vi "Add default dependencies.vi"(8 "error in (no error)":errorcluster, 11 "Targets in":refnum<class "Targets.lvclass">) -> (0 "error out":errorcluster, 3 "Targets out":refnum<class "Targets.lvclass">)   [LabVIEW 2013, in "PL Framework Configuration Tool.lvlib" / "Targets.lvclass"]
uses:
  Targets.lvclass
  Targets.lvclass/Targets.ctl
  TBM Configuration Node/deployment configuration.ctl
  TBM Configuration Node/TBM Configuration Node.lvclass
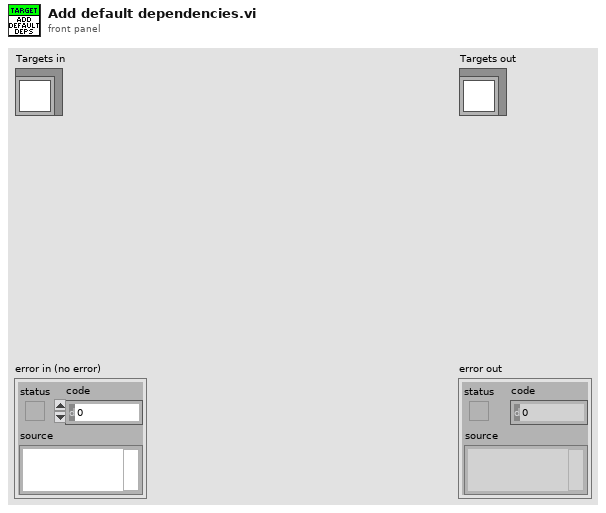
[diagram p1: front panel]
types:
  T1 = typedef "PL Framework Configuration Tool.lvlib/TBM Configuration Node.lvclass/deployment configuration.ctl" = cluster{"local path":path, "remote path (relative to root)":path}
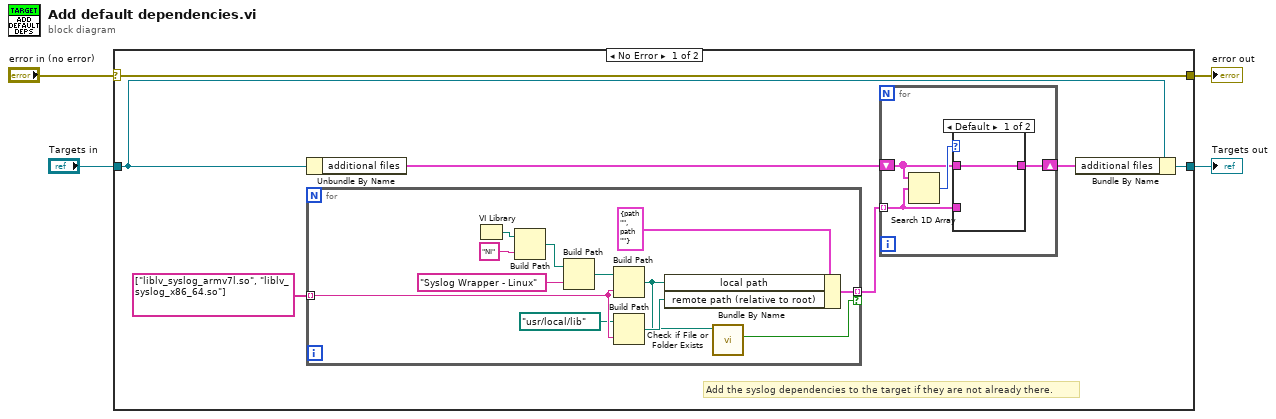
[diagram p0: block diagram]
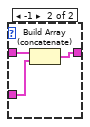
[diagram p2: hidden frame]
diagram:
  n1 = case shown="No Error" "error in (no error)" {
    selector: "error in (no error)" -> [w11 w33]
    tunnel: [w11 w33] -> w3
    tunnel: [w8 w32] -> w1
    tunnel: "Targets in" -> [w9 w32]
    frame No Error {
      # "Add the syslog dependencies to the target if they are not already there."
      n2 = Unbundle By Name(w9) -> ("additional files"=w7:T1[])
      n3 = for {
        tunnel: string[] ["liblv_syslog_armv7l.so", "liblv_syslog_x86_64.so"] -> [w24] mode=indexing
        tunnel: [w23] -> w6 mode=indexing if=w21
        n4 = VI Library() -> (path=w30:path)
        n5 = Build Path(base path=w30, name or relative path="NI") -> (appended path=w28:path)
        n6 = Build Path(base path=w28, name or relative path="Syslog Wrapper - Linux") -> (appended path=w26:path)
        n7 = Build Path(base path=w26, name or relative path=w24) -> (appended path=w22:path)
        n8 = Build Path(base path=path "/usr/local/lib", name or relative path=w24) -> (appended path=w25:path)
        n9 = Bundle By Name(cluster=T1 {"local path"=path "", "remote path (relative to root)"=path ""} ("deployment configuration"), "local path"=w22, "remote path (relative to root)"=w25) -> (w23:T1)
        n10 = call <vilib>:"Check if File or Folder Exists.vi"("path"=w22) -> ("file or folder exists?"=w21:bool)  [unwired: 8 in, 2 out]
      }
      n11 = for {
        shift-right: [w12] -> w5
        shift-left: w7 -> [w14]
        tunnel: w6 -> [w13] mode=indexing
        n12 = Search 1D Array(1D array=w14, element=w13) -> (index of element=w15:i32)  [unwired: 1 in]
        n13 = case shown="Default" w15 {
          tunnel: w14 -> [w16 w19]
          tunnel: w13 -> [_ w18]
          tunnel: [w16 w17] -> w12
          frame Default {
          }
          frame -1 {
            n14 = Build Array (concatenate)(w19, w18) -> (w17:T1[])
          }
        }
      }
      n15 = Bundle By Name(cluster=w9, "additional files"=w5) -> (w8:refnum<class "Targets.lvclass">)
    }
    frame Error {
    }
  }
  "error out" <- w3
  "Targets out" <- w1
